vi "VciDisplayError.vi"(3 "error in":errorcluster {"code" format="%.0x"}, 5 "HWND Parent":u32) -> ()   [LabVIEW 2011]
doc: "Shows a dialog box for the specified VCI error code."
uses:
  vcilva.dll
panel:
  in  "Caption":string
  out "error out":errorcluster {"code" format="%.0x"}
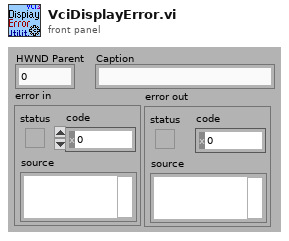
[diagram p1: front panel]
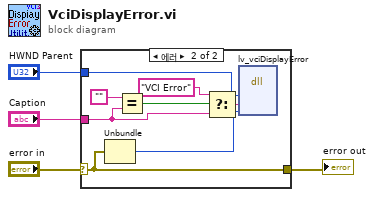
[diagram p0: block diagram]
diagram:
  n1 = case shown="에러" "error in" {
    selector: "error in" -> [w5 w13]
    tunnel: "HWND Parent" -> [_ w12]
    tunnel: [w5 w13] -> w4
    tunnel: "Caption" -> [_ w7]
    frame No Error {
    }
    frame Error {
      n2 = Unbundle(w13) -> ("code"=w11:i32)  [unwired: 2 out]
      n3 = Equal?(x="", y=w7) -> (x = y?=w9:bool)
      n4 = Select(t="VCI Error", s=w9, f=w7) -> (s? t:f=w8:string)
      n5 = dll-call lib="vcilva.dll" fn="lv_vciDisplayError"("hwndParent"=w12, "pszCaption"=w8, "hrError"=w11) -> ()  [unwired: 7 in, 2 out]
    }
  }
  "error out" <- w4
